vi "CRYGet Source Step from StepNo.vi"(10 "Protect?":bool, 11 "Step No.":i32) -> (3 "StepName":string)   [LabVIEW 2013]
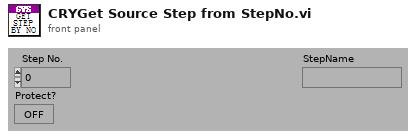
[diagram p1: front panel]
types:
  T1 = typedef "CRYStep.ctl" = cluster{"No.VI":i32, "Category":string, "StepName":string, "Seq setup flattened":string, "Comment":string, "Steps config.":bool[], "Jump config":i32[], "Start":dbl, "Increment":dbl, "Name":string, "Unit":string, "Y data":u16, "Y prefix":string, "Y dB ref":dbl, "Y unit":string, "Repeat State Array":cluster{"Start":dbl, "Increment":dbl, "Count":i32, "Num":i32}[]}
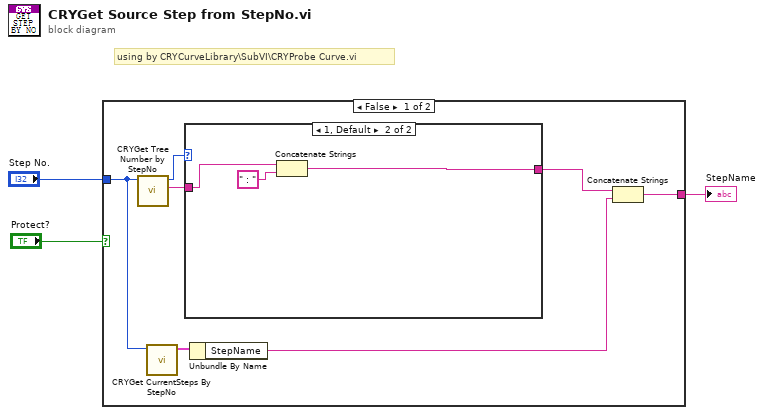
[diagram p0: block diagram]
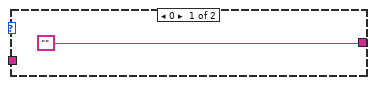
[diagram p2: hidden frame]
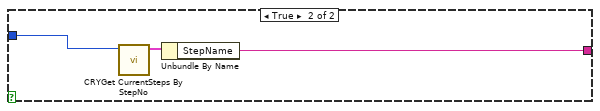
[diagram p3: hidden frame]
diagram:
  # "using by CRYCurveLibrary\\SubVI\\CRYProbe Curve.vi"
  n1 = case shown="False" "Protect?" {
    tunnel: [w8 w15] -> w1
    tunnel: "Step No." -> [w7 w16]
    frame False {
      n2 = call "CRYGet Tree Number by StepNo.vi"("Step Setup VI No"=w7) -> ("Number in SubSequence"=w4:string, "Number in Tree"=w6:i32)  [unwired: 9 in]
      n3 = call "CRYGet CurrentSteps By StepNo.vi"("Step Setup VI No"=w7) -> ("Step"=w10:T1)  [unwired: 8 in, 2 out]
      n4 = case shown="1, Default" w6 {
        tunnel: ["" w12] -> w5
        tunnel: w4 -> [_ w13]
        frame 0 {
        }
        frame 1, Default {
          n5 = Concatenate Strings(w13, " : " ("format string")) -> (w12:string)
        }
      }
      n6 = Unbundle By Name(w10) -> ("StepName"=w9:string)
      n7 = Concatenate Strings(w5, w9) -> (w8:string)
    }
    frame True {
      n8 = call "CRYGet CurrentSteps By StepNo.vi"("Step Setup VI No"=w16) -> ("Step"=w17:T1)  [unwired: 8 in, 2 out]
      n9 = Unbundle By Name(w17) -> ("StepName"=w15:string)
    }
  }
  "StepName" <- w1
